vi "Post.vi"(7 "Datum":refnum<class "Datum.lvclass">, 8 "Error In":errorcluster, 10 "Output In":string, 11 "Mock Render Variable Hook In":refnum<class "Mock Render Variable Hook.lvclass">) -> (0 "Error Out":errorcluster, 2 "Output Out":string, 3 "Mock Render Variable Hook Out":refnum<class "Mock Render Variable Hook.lvclass">)   [LabVIEW 2018, in "Tests.lvlib" / "Render.lvlib" / "Mock Render Variable Hook.lvclass"]
uses:
  Mock Render Variable Hook.lvclass
  src/Toolkit/Data/Datum/Datum.lvclass
  Mock Render Variable Hook.lvclass/Mock Render Variable Hook.ctl
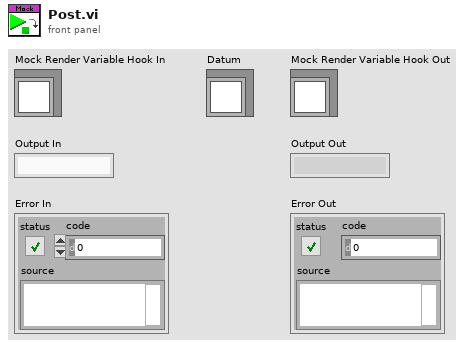
[diagram p1: front panel]
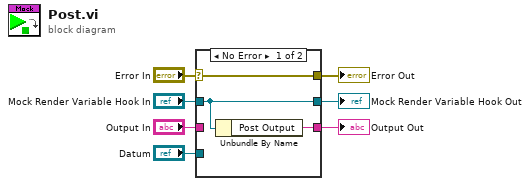
[diagram p0: block diagram]
diagram:
  n1 = case shown="No Error" "Error In" {
    selector: "Error In" -> [w10 w12]
    tunnel: [w10 w12] -> w6
    tunnel: "Output In" -> [_ w11]
    tunnel: "Mock Render Variable Hook In" -> [w8 w13]
    tunnel: [w8 w13] -> w3
    tunnel: "Datum" -> [_ _]
    tunnel: [w9 w11] -> w1
    frame No Error {
      n2 = Unbundle By Name(w8) -> ("Post Output"=w9:string)
    }
    frame Error {
    }
  }
  "Mock Render Variable Hook Out" <- w3
  "Error Out" <- w6
  "Output Out" <- w1
